vi "AvgPackGalvoData.vi"(8 "Laser Pulse":bool=TRUE, 9 "AcqStatusClock":u64, 11 "data in":T1={"channel 0"=[0, 0], "channel 1"=[0, 0], "channel 2"=[0, 0], "channel 3"=[0, 0], "channel 4"=[0, 0], "channel 5"=[0, 0], "channel 6"=[0, 0], "channel 7"=[0, 0]}) -> (0 "Data Valid Out":bool=TRUE, 3 "GalvoDataPack":u64[](array[numeric]))   [LabVIEW 2015]
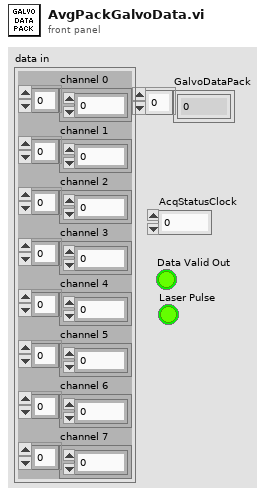
[diagram p1: front panel]
types:
  T1 = cluster{"channel 0":i16[], "channel 1":i16[], "channel 2":i16[], "channel 3":i16[], "channel 4":i16[], "channel 5":i16[], "channel 6":i16[], "channel 7":i16[]}
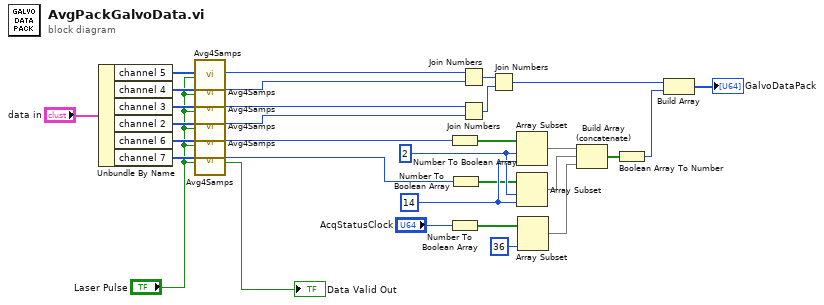
[diagram p0: block diagram]
diagram:
  w24 = 14 ("length")
  w23 = 2 ("index")
  n1 = Unbundle By Name("data in") -> ("channel 5"=w14:i16[], "channel 4"=w13:i16[], "channel 3"=w12:i16[], "channel 2"=w11:i16[], "channel 6"=w10:i16[], "channel 7"=w9:i16[])
  n2 = call "Avg4Samps.vi"("Input"=w14, "Start"="Laser Pulse") -> ("OuputAvg"=w7:i16)  [unwired: 16 in, 1 out]
  n3 = call "Avg4Samps.vi"("Input"=w13, "Start"="Laser Pulse") -> ("OuputAvg"=w6:i16)  [unwired: 16 in, 1 out]
  n4 = call "Avg4Samps.vi"("Input"=w12, "Start"="Laser Pulse") -> ("OuputAvg"=w5:i16)  [unwired: 16 in, 1 out]
  n5 = call "Avg4Samps.vi"("Input"=w11, "Start"="Laser Pulse") -> ("OuputAvg"=w4:i16)  [unwired: 16 in, 1 out]
  n6 = call "Avg4Samps.vi"("Input"=w10, "Start"="Laser Pulse") -> ("OuputAvg"=w3:i16)  [unwired: 16 in, 1 out]
  n7 = call "Avg4Samps.vi"("Input"=w9, "Start"="Laser Pulse") -> ("OuputAvg"=w2:i16, "Output Valid"=→"Data Valid Out":bool)  [unwired: 16 in]
  n8 = Number To Boolean Array(number=w3) -> (Boolean array=w20:bool[])
  n9 = Number To Boolean Array(number="AcqStatusClock") -> (Boolean array=w22:bool[])
  n10 = Number To Boolean Array(number=w2) -> (Boolean array=w21:bool[])
  n11 = Join Numbers(hi=w7, lo=w6) -> ((hi.lo)=w19:u32)
  n12 = Join Numbers(hi=w5, lo=w4) -> ((hi.lo)=w18:u32)
  n13 = Join Numbers(hi=w19, lo=w18) -> ((hi.lo)=w17:u64)
  n14 = Array Subset(array=w20, index=w23, length=w24) -> (w26:bool[])
  n15 = Array Subset(array=w21, index=w23, length=w24) -> (w27:bool[])
  n16 = Array Subset(array=w22, length=36) -> (w28:bool[])  [unwired: 1 in]
  n17 = Build Array (concatenate)(w26, w27, w28) -> (w30:bool[])
  n18 = Boolean Array To Number(Boolean array=w30) -> (number=w29:u64)
  n19 = Build Array(w17, w29) -> (→"GalvoDataPack":u64[])
